vi "Thingworx_ParseJSON.vi"(11 "Comm":T2) -> (2 "Table Control":string[][](table)=[["test", "test", "STRING"]], 3 "Data":T1(array[cluster]))   [LabVIEW 2020]
panel:
  out "Thing":string
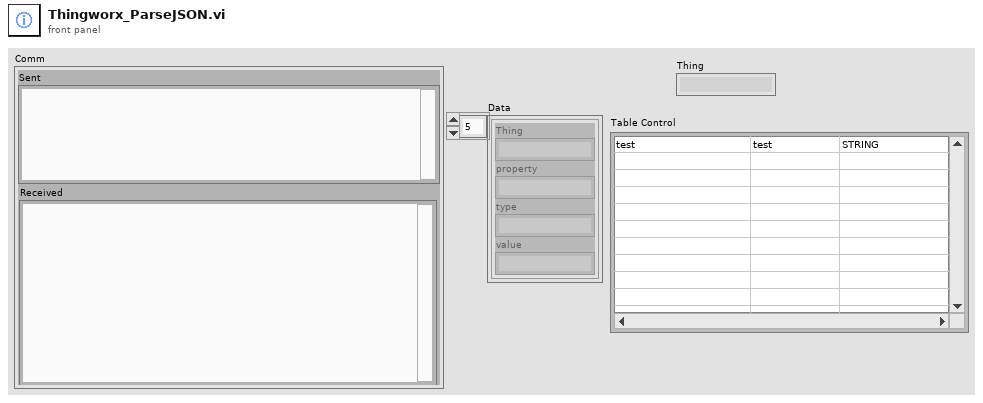
[diagram p1: front panel]
types:
  T1 = cluster{"Thing":string, "property":string, "type":string, "value":string}[]
  T2 = cluster{"url":string, "sent headers":string, "sent body":string, "headers":string, "body":string, "Sent":string, "Received":string}
  T3 = cluster{"Thing":string, "property":string, "type":string, "value":string}
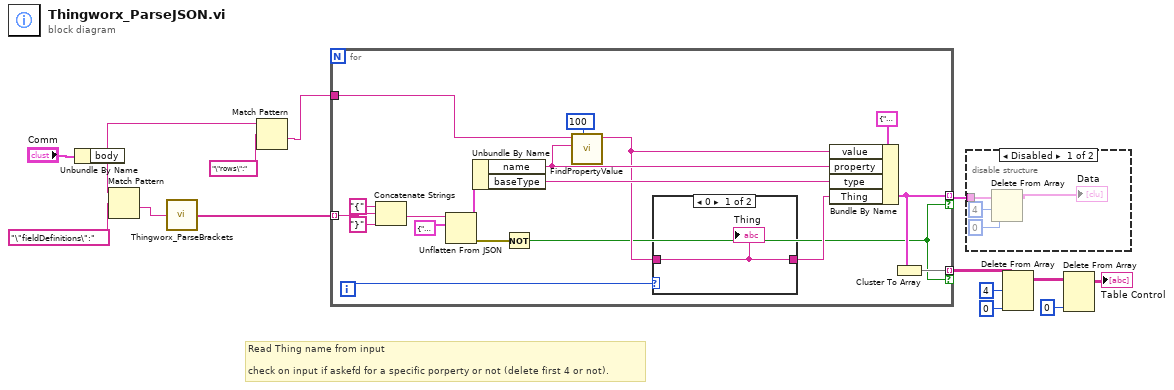
[diagram p0: block diagram]
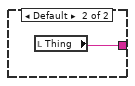
[diagram p3: hidden frame]
diagram:
  # "Read Thing name from input\n\ncheck on input if askefd for a specific porperty or not (delete first 4 or not)."
  n1 = Unbundle By Name("Comm") -> ("body"=w9:string)
  n2 = Match Pattern(string=w9, regular expression="\"fieldDefinitions\":") -> (after substring=w13:string)  [unwired: 1 in, 3 out]
  n3 = call "Thingworx_ParseBrackets.vi"("body"=w13) -> ("In Brackets"=w11:string[])
  n4 = Match Pattern(string=w9, regular expression="\"rows\":") -> (after substring=w8:string)  [unwired: 1 in, 3 out]
  n5 = for {
    tunnel: [w18] -> w7 mode=indexing if=w16
    tunnel: w11 -> [w28] mode=indexing
    tunnel: w8 -> [w23]
    tunnel: [w17] -> w4 mode=indexing if=w16
    i -> [w22]
    n6 = Concatenate Strings("{" ("string"), w28, "}" ("string")) -> (w32:string)
    n7 = Unflatten From JSON(JSON string=w32, type and defaults=cluster{"name":string, "baseType":string} {"name"="", "baseType"=""}) -> (value=w25:cluster{"name":string, "baseType":string}, error out=w26:errorcluster)  [unwired: 5 in]
    n8 = Unbundle By Name(w25) -> ("name"=w20:string, "baseType"=w24:string)
    n9 = Not(x=w26) -> (.not. x?=w16:bool)
    n10 = call "FindPropertyValue.vi"("max len"=100, "property"=w20, "rows"=w23) -> ("value"=w19:string)  [unwired: 8 in]
    n11 = case shown="0" w22 {
      tunnel: [w33 w34] -> w21
      tunnel: w19 -> [w33 _]
      frame 0 {
        "Thing" <- w33
      }
      frame Default {
        n12 = local read "Thing"() -> (w34:string)
      }
    }
    n13 = Bundle By Name(cluster=T3 {"Thing"="", "property"="", "type"="LONG", "value"=""} ("Property In"), "value"=w19, "property"=w20, "type"=w24, "Thing"=w21) -> (w18:T3)
    n14 = Cluster To Array(cluster=w18) -> (array=w17:string[])
  }
  n15 = disable-structure shown="Disabled" {
    disable-tunnel: w7 -> [w38 _]
    frame Disabled {
      n16 = Delete From Array(array=w38, length=4, index=0) -> (array with subset deleted=→"Data":T1)  [unwired: 1 out]
    }
    frame Enabled {
    }
  }
  n17 = Delete From Array(array=w4, length=4, index (row)=0 ("index")) -> (array with subset deleted=w3:string[][])  [unwired: 1 in, 1 out]
  n18 = Delete From Array(array=w3, index (col)=0 ("disabled index (col)")) -> (array with subset deleted=→"Table Control":string[][])  [unwired: 2 in, 1 out]
